vi "PRAT DO1.vi"(0 "VISA session":refnum<visa-resource-name>="MW100", 1 "Normally Closed Valve?":bool, 5 "PRAT Channels":T3, 7 "Valve Status":string, 11 "Error In":errorcluster) -> (4 "dup VISA session":refnum<visa-resource-name>, 6 "Send Command":string, 15 "Error":errorcluster)   [LabVIEW 2023]
uses:
  Type Definitions/PRAT Channel Settings.ctl
  Type Definitions/HEWH Normally Open Valve Control.ctl
  Type Definitions/HEWH Normally Closed Valve Control.ctl
panel:
  in  "Normally Closed Valve":T1
  in  "Normally Open Valve":T2
  # "PWR_MAIN: CLOSED = POWER OFF"
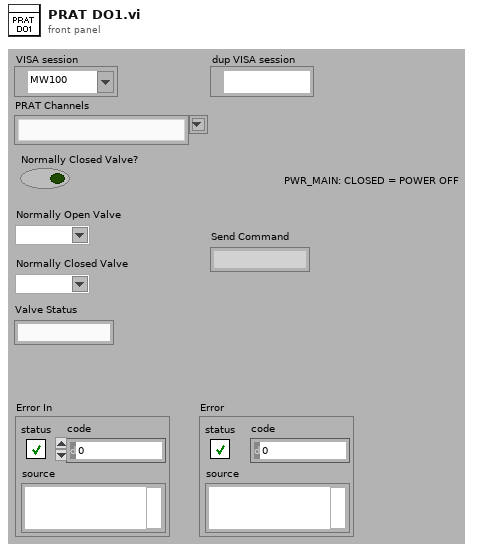
[diagram p1: front panel]
types:
  T1 = typedef "HEWH Normally Closed Valve Control.ctl" = string
  T2 = typedef "HEWH Normally Open Valve Control.ctl" = string
  T3 = typedef "PRAT Channel Settings.ctl" = string
  T4 = typedef "LVComboBoxStrsAndValuesArrayTypeDef.ctl" = cluster{"String":string, "Value":string}[]
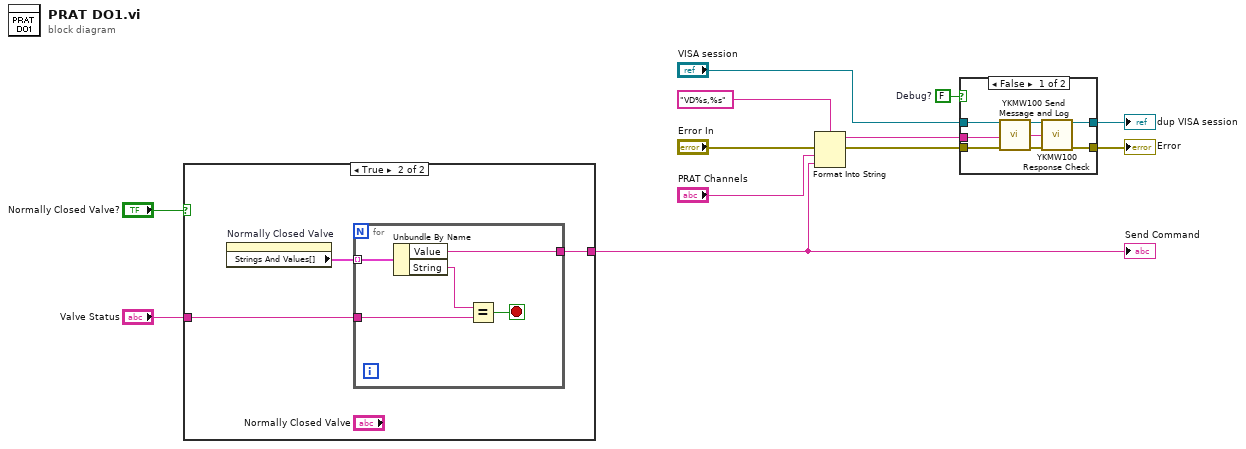
[diagram p0: block diagram]
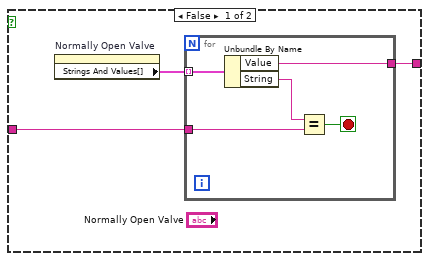
[diagram p3: hidden frame]
diagram:
  w3 = FALSE  # Debug?
  n1 = case shown="True" "Normally Closed Valve?" {
    tunnel: "Valve Status" -> [w13 w21]
    tunnel: [w14 w22] -> w1
    frame False {
      n2 = property on="Normally Open Valve" class="CmbBox (strict)"() -> ("Strings And Values[]"=w15:T4)  [unwired: 2 in, 2 out]
      n3 = for {
        tunnel: w15 -> [w20] mode=indexing
        tunnel: w13 -> [w18]
        tunnel: [w16] -> w14
        stop <- w17 stop-if-true
        n4 = Unbundle By Name(w20) -> ("Value"=w16:string, "String"=w19:string)
        n5 = Equal?(x=w19, y=w18) -> (x = y?=w17:bool)
      }
    }
    frame True {
      n6 = property on="Normally Closed Valve" class="CmbBox (strict)"() -> ("Strings And Values[]"=w23:T4)  [unwired: 2 in, 2 out]
      n7 = for {
        tunnel: w23 -> [w28] mode=indexing
        tunnel: w21 -> [w26]
        tunnel: [w24] -> w22
        stop <- w25 stop-if-true
        n8 = Unbundle By Name(w28) -> ("Value"=w24:string, "String"=w27:string)
        n9 = Equal?(x=w27, y=w26) -> (x = y?=w25:bool)
      }
    }
  }
  "Send Command" <- w1
  n10 = Format Into String(format string="VD%s,%s", error in="Error In", "PRAT Channels", w1) -> (resulting string=w8:string, error out=w9:errorcluster)  [unwired: 1 in]
  n11 = case shown="False" w3 {
    tunnel: "VISA session" -> [w36 w38]
    tunnel: [w35 w38] -> w10
    tunnel: w9 -> [w34 w37]
    tunnel: w8 -> [w33 _]
    tunnel: [w29 w37] -> w5
    frame False {
      n12 = call "YKMW100 Send Message and Log.vi"("VISA session"=w36, "Send Message (\"\")"=w33, "error in (no error)"=w34) -> ("dup VISA session"=w32:refnum<visa-resource-name>, "Read Buffer"=w30:string, "error out"=w31:errorcluster)  [unwired: 10 in]
      n13 = call "YKMW100 Response Check.vi"("VISA session"=w32, "Message In (\"\")"=w30, "error in (no error)"=w31) -> ("dup VISA session"=w35:refnum<visa-resource-name>, "error out"=w29:errorcluster)  [unwired: 8 in, 3 out]
    }
    frame True {
    }
  }
  "dup VISA session" <- w10
  "Error" <- w5
